vi "WPI_RelayOpen.vi"(8 "error in (no error)":errorcluster, 9 "Relay Direction":T1, 10 "Relay Channel":T2) -> (0 "error out":errorcluster, 3 "RelayDevRef":T3={"DevStatus"={"status"=FALSE, "code"=0, "source"=""}, "Relay Channel"=enum."Invalid", "Relay Direction"=enum."Both directions"})   [LabVIEW 2017]
doc: "Opens a reference to the relay you specify. You must open a reference before using any other VIs on this palette.\n\nThis software is licensed. Open the labview\\readme\\WPI Robotics Library Open Source License.txt file for more information."
uses:
  <vilib>/Rock Robotics/WPI/Relay/WPI_RelayDevRef.ctl
  <vilib>/Rock Robotics/SystemInterfaces/DIO/FPGA_DIORelayChannel.ctl
  <vilib>/Rock Robotics/WPI/Relay/WPI_RelayDirection.ctl
  <vilib>/Rock Robotics/WPI/Relay/WPI_RelayValue.ctl
  <vilib>/Rock Robotics/WPI/Relay/WPI_RelayCacheOp.ctl
  <vilib>/Rock Robotics/SystemInterfaces/NetworkCommunication/NetComm_UsageReport_ResourceType.ctl
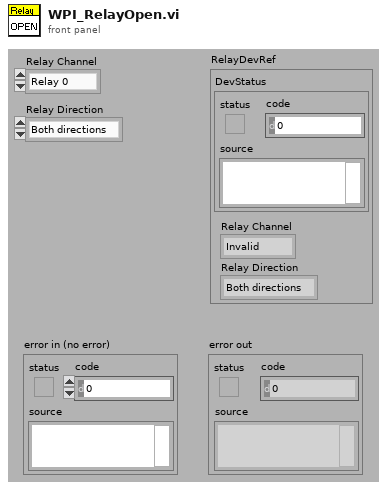
[diagram p1: front panel]
types:
  T1 = typedef "WPI_RelayDirection.ctl" = enum16{"Both directions", "Forward only", "Reverse only"}
  T2 = typedef "FPGA_DIORelayChannel.ctl" = enum8{"Relay 0", "Relay 1", "Relay 2", "Relay 3", "Invalid"}
  T3 = typedef "WPI_RelayDevRef.ctl" = cluster{"DevStatus":errorcluster, "Relay Channel":T2, "Relay Direction":T1}
  T4 = typedef "WPI_RelayCacheOp.ctl" = enum16{"Acquire", "Release", "Status"}
  T5 = typedef "WPI_RelayValue.ctl" = enum16{"Off", "On", "Forward", "Reverse"}
  T6 = typedef "NetComm_UsageReport_ResourceType.ctl" = enum8{"Controller", "Module", "Language", "CANPlugin", "Accelerometer", "ADXL345", "AnalogChannel", "AnalogTrigger", "AnalogTriggerOutput", "CANJaguar", "Compressor", "Counter", "Dashboard", "DigitalInput", "DigitalOutput", "DriverStationCIO", "DriverStationEIO", "DriverStationLCD", "Encoder", "GearTooth", "Gyro", "I2C", "Framework", "Jaguar", "Joystick", "Kinect", "KinectStick", "PIDController", "Preferences", "PWM", "Relay", "RobotDrive", "SerialPort", "Servo", "Solenoid", "SPI", "Task", "Ultrasonic", "Victor", "Button", "Command", "AxisCamera", "PCVideoServer", "SmartDashboard", "Talon", "HiTechnicColorSensor", "HiTechnicAccel", "HiTechnicCompass", "SRF08", "AnalogOutput", "Victor SP", "Talon SRX", "CAN Talon SRX", "ADXL362 Accel", "ADXRS450 Gyro", "Rev SPARK", "Mindsensors SD540", "Digital Filter", "ADIS16448", "PDP", "PCM", "PigeonIMU", "Nidec Brushless", "CTRE CANifier", "CTRE Future 0", "CTRE Future 1", "CTRE Future 2", "CTRE Future 3", "CTRE Future 4", "CTRE Future 5", "CTRE Future 6"}
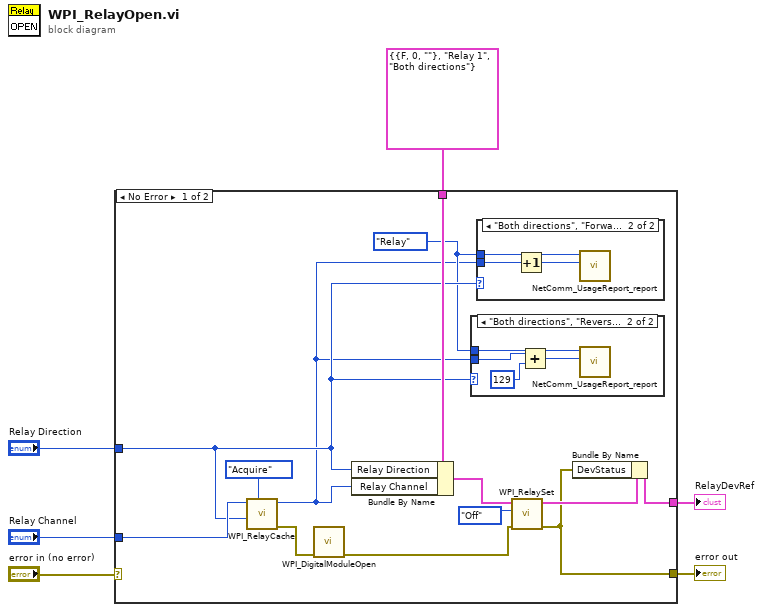
[diagram p0: block diagram]
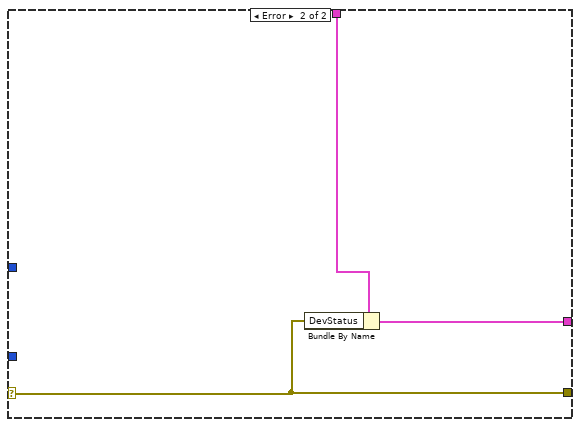
[diagram p4: hidden frame]
diagram:
  n1 = case shown="No Error" "error in (no error)" {
    selector: "error in (no error)" -> [_ w29]
    tunnel: "Relay Channel" -> [w17 _]
    tunnel: [w7 w27] -> w5
    tunnel: [w11 w29] -> w4
    tunnel: T3 {"DevStatus"={"status"=FALSE, "code"=0, "source"=""}, "Relay Channel"=enum."Relay 1", "Relay Direction"=enum."Both directions"} ("RelayDevRef") -> [w19 w28]
    tunnel: "Relay Direction" -> [w10 _]
    frame No Error {
      w9 = NetComm_UsageReport_ResourceType."Relay" ("Resource Type")
      n2 = call <vilib>:"WPI_RelayCache.vi"("Operation"=WPI_RelayCacheOp."Acquire", "RelayDirection"=w10, "RelayChannelIn"=w17) -> ("error out"=w14:errorcluster, "RelayChannelOut"=w8:T2)  [unwired: 2 in, 5 out]
      n3 = call <vilib>:"WPI_DigitalModuleOpen.vi"("error in (no error)"=w14) -> ("error out"=w13:errorcluster)  [unwired: 1 in, 9 out]
      n4 = Bundle By Name(cluster=w19, "Relay Direction"=w10, "Relay Channel"=w8) -> (w15:T3)
      n5 = case shown="\"Both directions\", \"Reverse only\"" w10 {
        tunnel: w9 -> [_ w23]
        tunnel: w8 -> [_ w22]
        frame Default {
        }
        frame "Both directions", "Reverse only" {
          n6 = Add(x=w22, y=129) -> (x+y=w20:i32)
          n7 = call <vilib>:"NetComm_UsageReport_report.vi"("Instance Number"=w20, "Resource Type"=w23) -> ()  [unwired: 10 in]
        }
      }
      n8 = case shown="\"Both directions\", \"Forward only\"" w10 {
        tunnel: w9 -> [_ w26]
        tunnel: w8 -> [_ w25]
        frame Default {
        }
        frame "Both directions", "Forward only" {
          n9 = Increment(x=w25) -> (x+1=w24:T2)
          n10 = call <vilib>:"NetComm_UsageReport_report.vi"("Instance Number"=w24, "Resource Type"=w26) -> ()  [unwired: 10 in]
        }
      }
      n11 = call <vilib>:"WPI_RelaySet.vi"("error in (no error)"=w13, "RelayValue"=WPI_RelayValue."Off", "RelayDevRef"=w15) -> ("error out"=w11:errorcluster, "RelayDevRef"=w12:T3)  [unwired: 7 out]
      n12 = Bundle By Name(cluster=w12, "DevStatus"=w11) -> (w7:T3)
    }
    frame Error {
      n13 = Bundle By Name(cluster=w28, "DevStatus"=w29) -> (w27:T3)
    }
  }
  "error out" <- w4
  "RelayDevRef" <- w5
